vi "LabsqlInsert.vi"(2 "Cluster":cluster{"实验ID筛选":string, "应变值筛选":string}, 3 "数据库配置":T1, 4 "存入的应变值":dbl) -> (0 "数组 - 字符串":string[][](array[string]), 1 "error out":errorcluster)   [LabVIEW 2019]
doc: "This example opens a connection to a database specified by the Connection string (replace the DNS name with your database) inserts a new row into the table \"myOtherTable\" (replace the SQL string with your own SQL query)."
panel:
  out "select":string
  out "insert":string
  # "应变数据："
  # "数据链接："
  # "实验标签："
  # "列名3："
  # "列名2："
  # "列名1："
  # "写入表名："
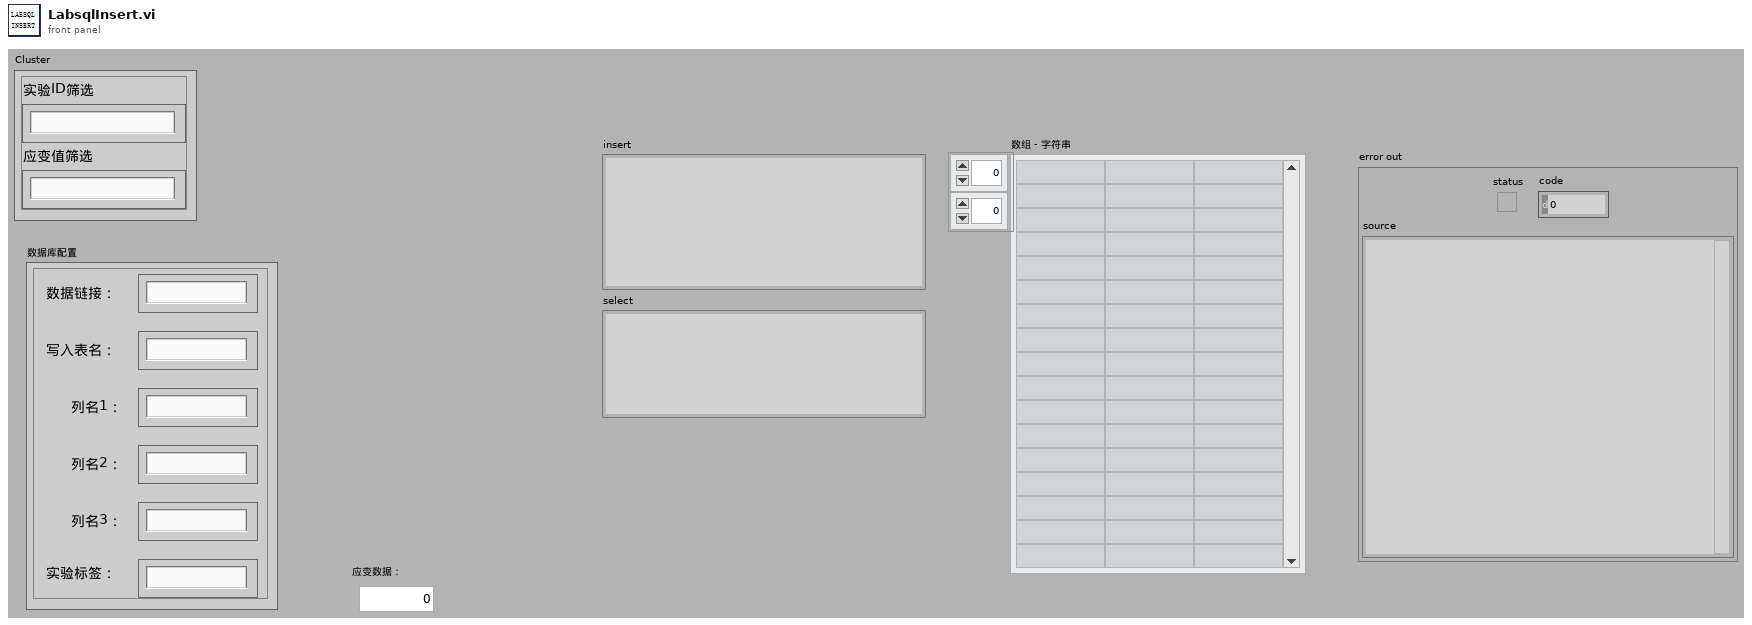
[diagram p1: front panel]
types:
  T1 = cluster{"String":string, "String 2":string, "String 3":string, "String 4":string, "String 5":string, "String 6":string}
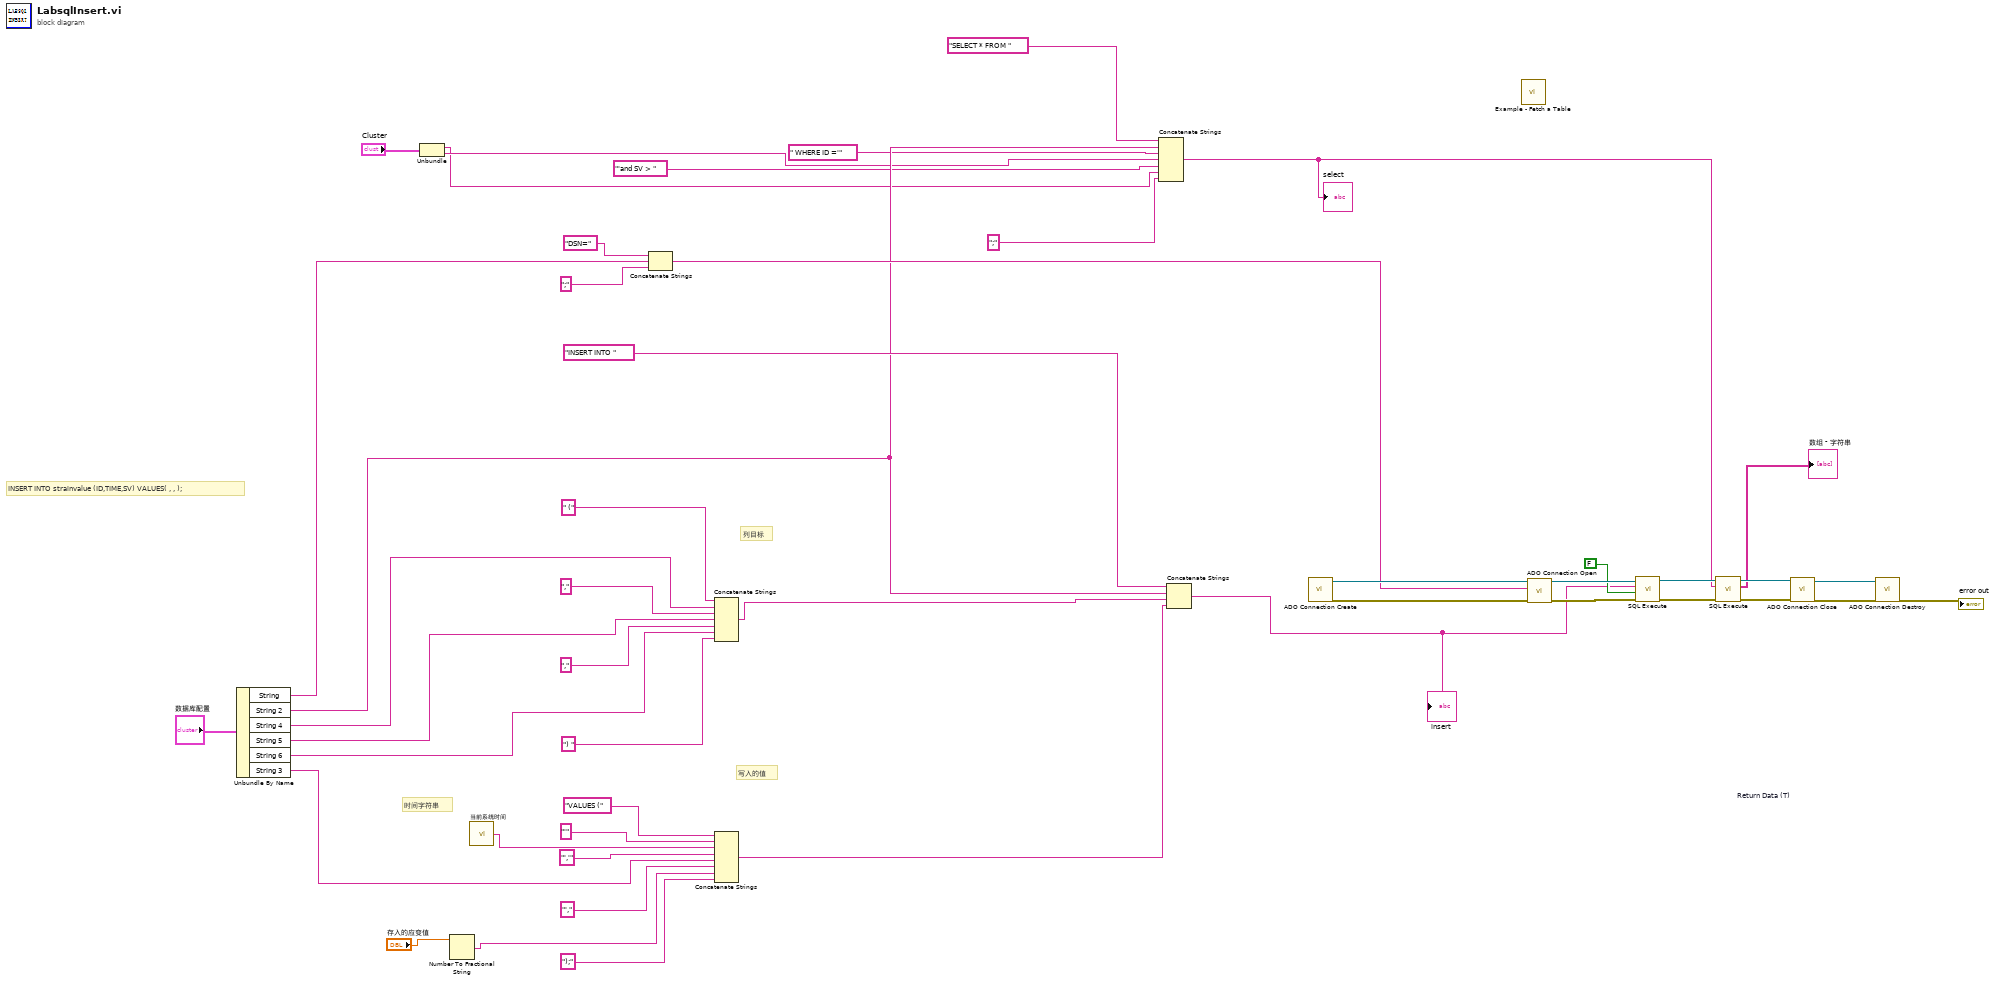
[diagram p0: block diagram]
diagram:
  w40 = FALSE  # Return Data (T)
  # "时间字符串"
  # "写入的值"
  # "列目标"
  # "INSERT INTO strainvalue (ID,TIME,SV) VALUES( , , );"
  n1 = Unbundle By Name("数据库配置") -> ("String"=w37:string, "String 2"=w19:string, "String 4"=w24:string, "String 5"=w23:string, "String 6"=w22:string, "String 3"=w8:string)
  n2 = Unbundle("Cluster") -> ("实验ID筛选"=w5:string, "应变值筛选"=w6:string)
  n3 = Number To Fractional String(number="存入的应变值") -> (F-format string=w3:string)  [unwired: 3 in]
  n4 = call "当前系统时间.vi"() -> ("日期/时间字符串"=w9:string)
  n5 = Concatenate Strings("DSN=", w37, ";" ("字符串")) -> (w21:string)
  n6 = Concatenate Strings(" (" ("字符串"), w24, "," ("字符串"), w23, "," ("字符串"), w22, ") " ("字符串")) -> (w31:string)
  n7 = Concatenate Strings("VALUES (" ("字符串"), "'" ("字符串"), w9, "','" ("字符串"), w8, "'," ("字符串"), w3, ");" ("字符串")) -> (w25:string)
  n8 = Concatenate Strings("SELECT * FROM " ("字符串"), w19, " WHERE ID ='" ("字符串"), w6, "'and SV > " ("字符串"), w5, ";" ("字符串")) -> (w11:string)
  "select" <- w11
  n9 = Concatenate Strings("INSERT INTO " ("字符串"), w19, w31, w25) -> (w35:string)
  "insert" <- w35
  n10 = call <userlib>:"ADO Connection Create.vi"() -> ("error out"=w46:errorcluster, "ADODB._Connection Out"=w47:refnum<k7>)  [unwired: 10 in]
  n11 = call <userlib>:"Example - Fetch a Table.vi"() -> ()  [unwired: 1 in]
  n12 = call <userlib>:"ADO Connection Open.vi"("error in (no error)"=w46, "ConnectionString"=w21, "ADODB._Connection In"=w47) -> ("error out"=w44:errorcluster, "ADODB._Connection Out"=w45:refnum<k7>)  [unwired: 7 in]
  n13 = call <userlib>:"SQL Execute.vi"("error in (no error)"=w44, "Return Data (T)"=w40, "Command Text"=w35, "ADODB._Connection In"=w45) -> ("error out"=w17:errorcluster, "ADODB._Connection Out"=w18:refnum<k7>)  [unwired: 4 in, 2 out]
  n14 = call <userlib>:"SQL Execute.vi"("error in (no error)"=w17, "Command Text"=w11, "ADODB._Connection In"=w18) -> ("error out"=w15:errorcluster, "Data"=→"数组 - 字符串":string[][], "ADODB._Connection Out"=w16:refnum<k7>)  [unwired: 5 in, 1 out]
  n15 = call <userlib>:"ADO Connection Close.vi"("error in (no error)"=w15, "ADODB._Connection In"=w16) -> ("error out"=w43:errorcluster, "ADODB._Connection Out"=w42:refnum<k7>)  [unwired: 8 in]
  n16 = call <userlib>:"ADO Connection Destroy.vi"("error in (no error)"=w43, "ADODB._Connection In"=w42) -> ("error out"=→"error out":errorcluster)  [unwired: 9 in]
